vi "RichToFlatnidaqmx_grpc_GetChanAttributeStringResponse.vi"(5 "OutputClusterType":T1, 11 "InputCluster":T2) -> (3 "OutputCluster":T1)   [LabVIEW 2021, in "NI_DAQmx_client.lvlib"]
uses:
  NI_DAQmx_client.lvlib
  nidaqmx_grpc_GetChanAttributeStringResponse_Flat.ctl
  nidaqmx_grpc_GetChanAttributeStringResponse.ctl
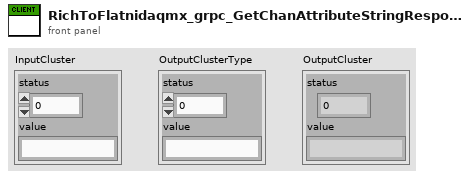
[diagram p1: front panel]
types:
  T1 = typedef "NI_DAQmx_client.lvlib/nidaqmx_grpc_GetChanAttributeStringResponse_Flat.ctl" = cluster{"status":i32, "value":string}
  T2 = typedef "NI_DAQmx_client.lvlib/nidaqmx_grpc_GetChanAttributeStringResponse.ctl" = cluster{"status":i32, "value":string}
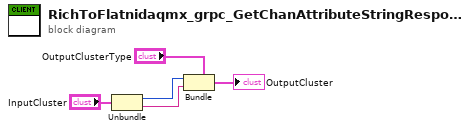
[diagram p0: block diagram]
diagram:
  n1 = Unbundle "Unbundle"("InputCluster") -> ("status"=w2:i32, "value"=w1:string)
  n2 = Bundle "Bundle"(cluster="OutputClusterType", "status"=w2, "value"=w1) -> (→"OutputCluster":T1)
